vi "TDTSyn-Wait For Block.vi"(0 "IP Address":string, 5 "Port":i32, 9 "Timeout (s)":i32=10, 11 "error in (no error)":errorcluster) -> (15 "error out":errorcluster)   [LabVIEW 2020]
panel:
  out "block name":string
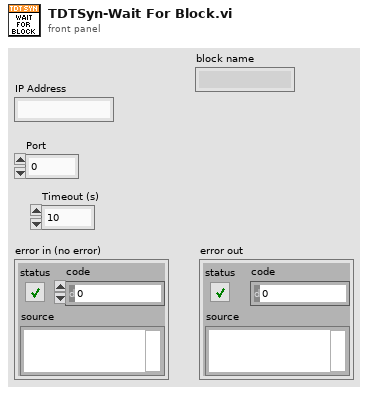
[diagram p1: front panel]
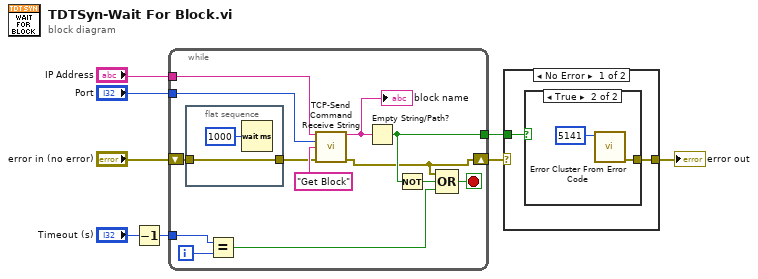
[diagram p0: block diagram]
diagram:
  n1 = Decrement(x="Timeout (s)") -> (x-1=w4:i32)
  n2 = while {
    shift-right: [w12] -> w3
    shift-left: "error in (no error)" -> [w10]
    tunnel: "IP Address" -> [w20]
    tunnel: "Port" -> [w21]
    tunnel: [w16] -> w1
    tunnel: w4 -> [w11]
    i -> [w17]
    stop <- w13 stop-if-true
    n3 = flat-sequence {
      tunnel: w10 -> [w23]
      tunnel: [w23] -> w9
      frame #0 {
        n4 = Wait (ms)(milliseconds to wait=u32 1000) -> ()  [unwired: 1 out]
      }
    }
    n5 = Equal?(x=w11, y=w17) -> (x = y?=w14:bool)
    n6 = call "TCP-Send Command Receive String.vi"("PXI Address"=w20, "Port"=w21, "Command"="Get Block", "error in (no error)"=w9) -> ("data"=w18:string, "error out"=w12:errorcluster)  [unwired: 9 in, 1 out]
    "block name" <- w18
    n7 = Empty String/Path?(string/path=w18) -> (empty?=w16:bool)
    n8 = Not(x=w16) -> (.not. x?=w15:bool)
    n9 = Compound Arithmetic op=OR(w12, w15, w14) -> (w13:bool)
  }
  n10 = case shown="No Error" w3 {
    selector: w3 -> [_ w28]
    tunnel: [w24 w28] -> w2
    tunnel: w1 -> [w25 _]
    frame No Error {
      n11 = case shown="True" w25 {
        tunnel: [_ w27] -> w24
        frame False {
        }
        frame True {
          n12 = call <vilib>:"Error Cluster From Error Code.vi"("error code (0)"=5141) -> ("error out"=w27:errorcluster)  [unwired: 8 in]
        }
      }
    }
    frame Error {
    }
  }
  "error out" <- w2
